vi "Initialize Osciloscope.vi"(8 "error in (no error)":errorcluster, 10 "Initialize--cluster":T1={"TEKTRONIX-INITIALIZE"={"ID Query? (T: Yes)"=TRUE, "Reset? (T: Yes)"=TRUE, "Serial-Configuration"={"Baud Rate"=9600, "Parity"=0, "Stop Bits"=10, "Flow Control"=2}}, "EDU-X-1200A- INITIALIZE"={"Reset (True)"=TRUE, "ID Query (True)"=TRUE}} {"TEKTRONIX-INITIALIZE"."Serial-Configuration"."Flow Control" items=["None", "XON/XOFF", "RTS/CTS", "XON/XOFF & RTS/CTS", "DTR/DSR", "XON/XOFF & DTR/DSR"]; "TEKTRONIX-INITIALIZE"."Serial-Configuration"."Stop Bits" items=["1.0"=10, "1.5"=15, "2.0"=20]; "TEKTRONIX-INITIALIZE"."Serial-Configuration"."Parity" items=["None", "Odd", "Even", "Mark", "Space"]; "TEKTRONIX-INITIALIZE"."Serial-Configuration"."Baud Rate" items=["300"=300, "600"=600, "1200"=1200, "2400"=2400, "4800"=4800, "9600"=9600, "19200"=19200]}, 11 "Tektronicks in":refnum<class "Tektronicks.lvclass">) -> (0 "error out":errorcluster, 3 "Tektronicks out":refnum<class "Tektronicks.lvclass">)   [LabVIEW 2020, in "Tektronicks.lvclass"]
uses:
  Tektronicks.lvclass
  TypeDefs/InitializeOsciloscope--cluster.ctl
  Tektronicks.lvclass/Tektronicks.ctl
  <instrlib>/Tektronix TDS 200 1000 2000 Series/Tektronix TDS 200 1000 2000 Series.lvlib
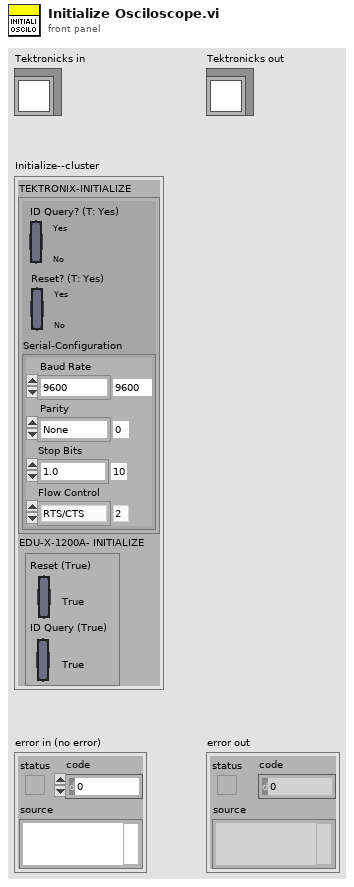
[diagram p1: front panel]
types:
  T1 = typedef "InitializeOsciloscope--cluster.ctl" = cluster{"TEKTRONIX-INITIALIZE":cluster{"ID Query? (T: Yes)":bool, "Reset? (T: Yes)":bool, "Serial-Configuration":cluster{"Baud Rate":u32, "Parity":u16, "Stop Bits":u16, "Flow Control":u16}}, "EDU-X-1200A- INITIALIZE":cluster{"Reset (True)":bool, "ID Query (True)":bool}}
  T2 = cluster{"Baud Rate":u32, "Parity":u16, "Stop Bits":u16, "Flow Control":u16}
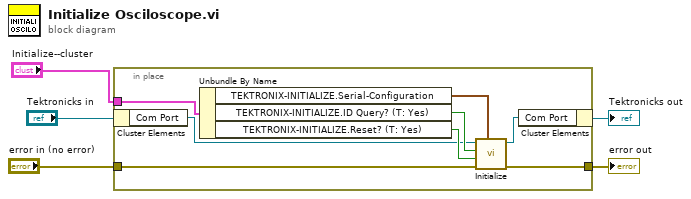
[diagram p0: block diagram]
diagram:
  n1 = in-place {
    in-place-border: "Initialize--cluster" -> [w13]
    in-place-border: "error in (no error)" -> [w9]
    in-place-border: [w8] -> w1
    n2 = in-place-cluster #1("Tektronicks in") -> ("Com Port"=w7:refnum<visa-resource-name>)
    n3 = Unbundle By Name(w13) -> ("TEKTRONIX-INITIALIZE.Serial-Configuration"=w12:T2, "TEKTRONIX-INITIALIZE.ID Query? (T: Yes)"=w11:bool, "TEKTRONIX-INITIALIZE.Reset? (T: Yes)"=w10:bool)
    n4 = call <instrlib>:"Initialize.vi"("Serial Configuration"=w12, "error in (no error)"=w9, "Reset? (T: Yes)"=w10, "ID Query? (T: Yes)"=w11, "VISA resource name"=w7) -> ("error out"=w8:errorcluster, "VISA resource name out"=w6:refnum<visa-resource-name>)  [unwired: 5 in]
    n5 = in-place-cluster #1("Com Port"=w6) -> (→"Tektronicks out":refnum<class "Tektronicks.lvclass">)
  }
  "error out" <- w1
